vi "Clear Setpoints.vi"(8 "error in (no error)":errorcluster, 11 "Model in":refnum<class "Model.lvclass">) -> (0 "error out":errorcluster, 3 "Model out":refnum<class "Model.lvclass">)   [LabVIEW 2016]
uses:
  Typedefs/ActuatorSetPoints.ctl
  Model.lvclass
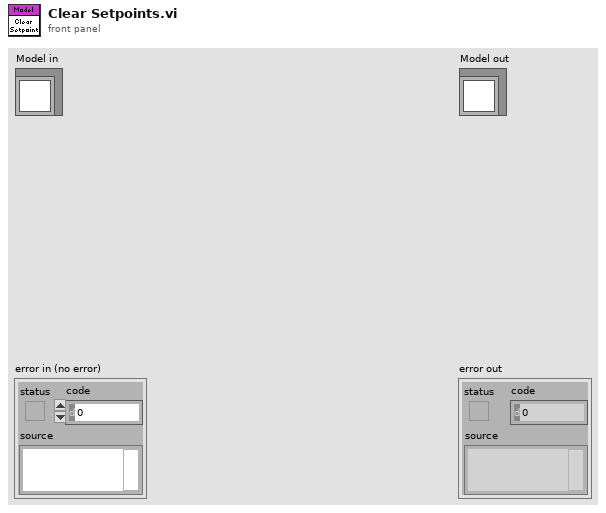
[diagram p1: front panel]
types:
  T1 = typedef "ActuatorSetPoints.ctl" = cluster{"Axial Force":dbl, "Lateral Force":dbl, "FC1 Force":dbl, "FC2 Force":dbl}
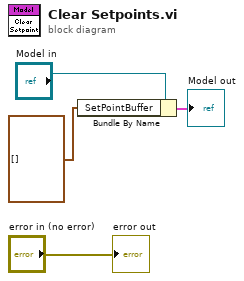
[diagram p0: block diagram]
diagram:
  n1 = Bundle By Name(cluster="Model in", "SetPointBuffer"=T1[] []) -> (→"Model out":cluster{})
  "error out" <- "error in (no error)"
